vi "open_python_from_text.vi"(8 "error in (no error)":errorcluster, 11 "Python Function:":string) -> (0 "error out":errorcluster, 1 "function name":string, 2 "module path":path, 3 "Refnum out":refnum<k35>)   [LabVIEW 2022 SP3]
uses:
  <vilib>/regexp/Match Regular Expression.xnode
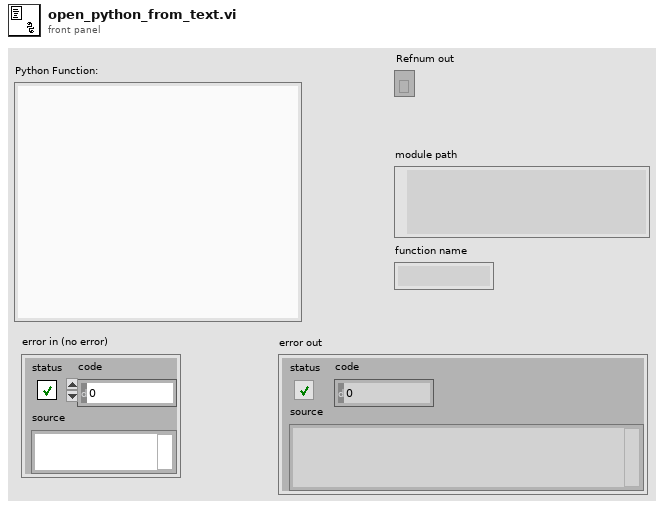
[diagram p1: front panel]
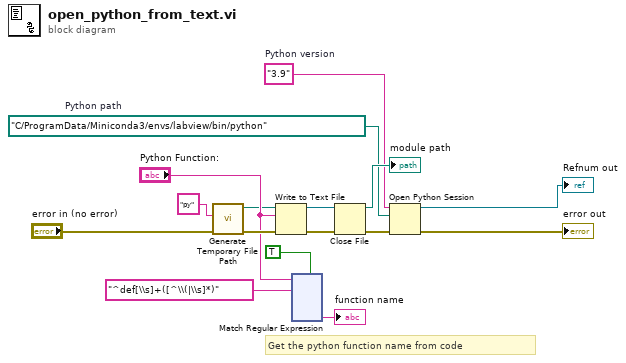
[diagram p0: block diagram]
diagram:
  w3 = path "C:/ProgramData/Miniconda3/envs/labview/bin/python"  # Python path
  w2 = "3.9"  # Python version
  # "Get the python function name from code"
  n1 = call <vilib>:"Generate Temporary File Path.vi"("error in (no error)"="error in (no error)", "Temporary File Extension (tmp)"="py") -> ("error out"=w14:errorcluster, "Unique Temporary File Path"=w8:path)  [unwired: 8 in]
  n2 = Write to Text File(file (use dialog)=w8, text="Python Function:", error in=w14) -> (refnum out=w9:refnum<file>, error out=w11:errorcluster)  [unwired: 1 in, 1 out]
  n3 = xnode "Match Regular Expression"("input string"="Python Function:", "regular expression"="^def[\\s]+([^\\(|\\s]*)", "multiline? (F)"=TRUE) -> ("submatch 1"=→"function name":string)  [unwired: 3 in, 5 out]
  n4 = Close File(refnum=w9, error in=w11) -> (path=→"module path":path, error out=w15:errorcluster)
  n5 = Open Python Session(python version=w2, python path=w3, 3:w15) -> (session out=→"Refnum out":refnum<k35>, error out=→"error out":errorcluster)
